vi "Load to memory.vi"(0 "Document in":refnum<class "Document.lvclass">, 5 "Path":path, 7 "Batch File":path, 11 "error in (no error)":errorcluster) -> (4 "Document out":refnum<class "Document.lvclass">, 6 "Names[]":string[](array[string]), 8 "Child Window Data":T1, 15 "error out":errorcluster)   [LabVIEW 2016, in "Document.lvclass"]
uses:
  Document.lvclass
  Private/Child Window Data.ctl
  LV MDI.lvclass
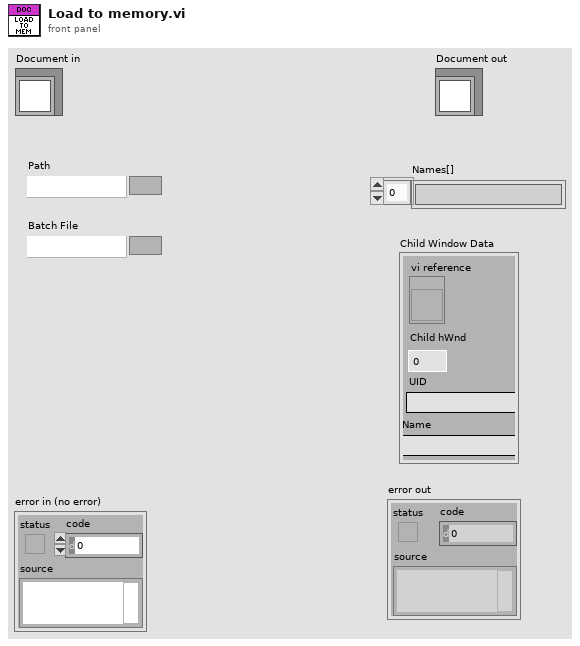
[diagram p1: front panel]
types:
  T1 = typedef "LV MDI.lvclass/Child Window Data.ctl" = cluster{"Child hWnd":u32, "UID":string, "vi reference":refnum<vi>, "Name":string}
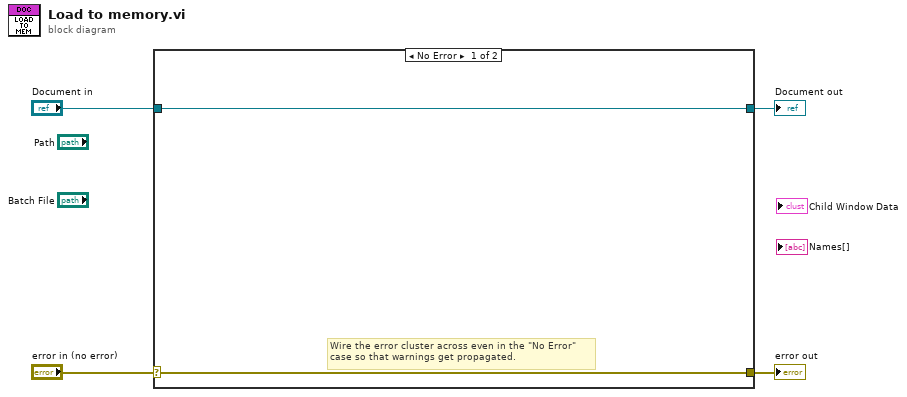
[diagram p0: block diagram]
diagram:
  n1 = case shown="No Error" "error in (no error)" {
    selector: "error in (no error)" -> [w5 w8]
    tunnel: [w5 w8] -> w3
    tunnel: [w6 w7] -> w1
    tunnel: "Document in" -> [w6 w7]
    frame No Error {
      # "Wire the error cluster across even in the \"No Error\"\ncase so that warnings get propagated."
    }
    frame Error {
    }
  }
  "error out" <- w3
  "Document out" <- w1
